vi "DrawRectangle.vi"() -> ()   [LabVIEW 2020]
panel:
  in  "path to BMP file":path
  out "2D Picture":picture
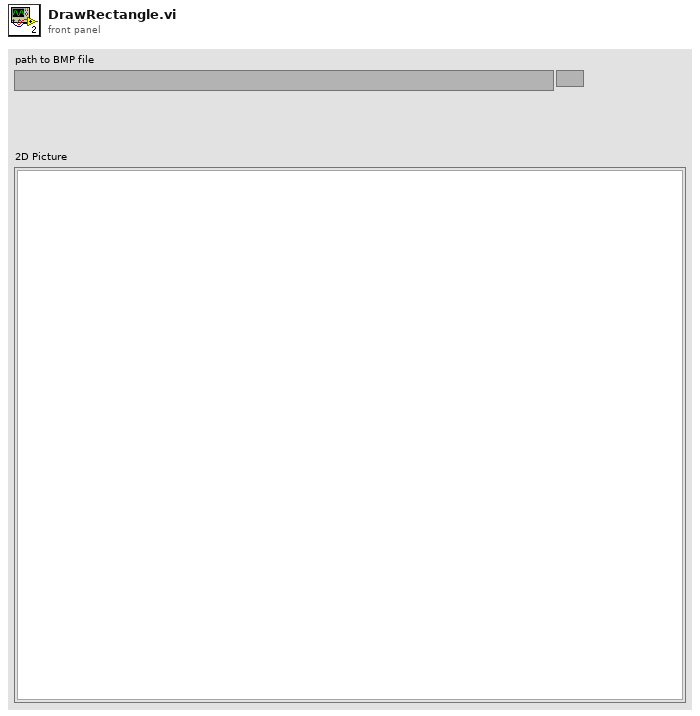
[diagram p1: front panel]
types:
  T1 = typedef "imagedata.ctl" = cluster{"image type":i32, "image depth":i32, "image":u8[], "mask":u8[], "colors":u32[], "Rectangle":cluster{"left":i16, "top":i16, "right":i16, "bottom":i16}}
  T2 = cluster{"Width":i16, "Style":enum32{"Solid", "Dash", "Dot", "DashDot", "DashDotDot"}}
  T3 = cluster{"left":i16, "top":i16, "right":i16, "bottom":i16}
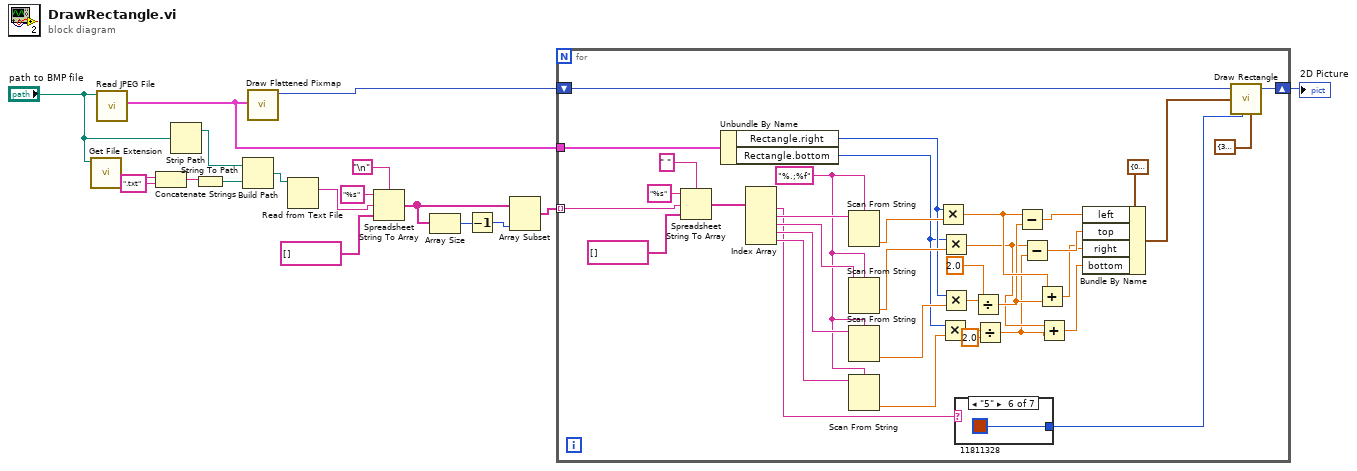
[diagram p0: block diagram]
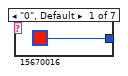
[diagram p2: hidden frame]
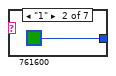
[diagram p3: hidden frame]
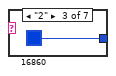
[diagram p4: hidden frame]
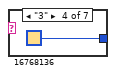
[diagram p5: hidden frame]
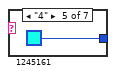
[diagram p6: hidden frame]
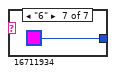
[diagram p7: hidden frame]
diagram:
  n1 = call <vilib>:"Get File Extension.vi"("file"="path to BMP file") -> ("filename without extension"=w18:string)  [unwired: 6 in, 4 out]
  n2 = call <vilib>:"Read JPEG File.vi"("path to JPEG file"="path to BMP file") -> ("image data"=w9:T1)  [unwired: 8 in, 2 out]
  n3 = Concatenate Strings(w18, ".txt" ("string")) -> (w16:string)
  n4 = Strip Path(path="path to BMP file") -> (stripped path=w13:path)  [unwired: 1 out]
  n5 = String To Path(string=w16) -> (path=w15:path)
  n6 = Build Path(base path=w13, name or relative path=w15) -> (appended path=w12:path)
  n7 = call <vilib>:"Draw Flattened Pixmap.vi"("image data"=w9) -> ("new picture"=w10:picture)  [unwired: 8 in]
  n8 = Read from Text File(file (use dialog)=w12) -> (text=w6:string)  [unwired: 3 in, 3 out]
  n9 = Spreadsheet String To Array(delimiter (Tab)="\n", format string="%s", spreadsheet string=w6, array type (2D Dbl)=string[] []) -> (array=w3:string[])
  n10 = Array Size(array=w3) -> (size(s)=w2:i32)
  n11 = Decrement(x=w2) -> (x-1=w1:i32)
  n12 = Array Subset(array=w3, length=w1) -> (w4:string[])  [unwired: 1 in]
  n13 = for {
    tunnel: w9 -> [w34]
    shift-right: [w39] -> w11
    shift-left: w10 -> [w35]
    tunnel: w4 -> [w20] mode=indexing
    w46 = "%.;%f" ("format string")
    n14 = Spreadsheet String To Array(delimiter (Tab)=" ", format string="%s", spreadsheet string=w20, array type (2D Dbl)=string[] []) -> (array=w52:string[])
    n15 = Unbundle By Name(w34) -> ("Rectangle.right"=w41:i16, "Rectangle.bottom"=w40:i16)
    n16 = Index Array(array=w52) -> (element #1=w19:string, element #2=w50:string, element #3=w47:string, element #4=w48:string, element #5=w49:string)  [unwired: 5 in]
    n17 = Scan From String(format string=w46, input string=w50) -> (output 1=w43:dbl)  [unwired: 3 in, 3 out]
    n18 = Scan From String(format string=w46, input string=w47) -> (output 1=w42:dbl)  [unwired: 3 in, 3 out]
    n19 = Scan From String(format string=w46, input string=w48) -> (output 1=w44:dbl)  [unwired: 3 in, 3 out]
    n20 = Scan From String(format string=w46, input string=w49) -> (output 1=w45:dbl)  [unwired: 3 in, 3 out]
    n21 = Multiply(x=w41, y=w43) -> (x*y=w27:dbl)
    n22 = Multiply(x=w40, y=w45) -> (x*y=w32:dbl)
    n23 = Multiply(x=w40, y=w42) -> (x*y=w24:dbl)
    n24 = Multiply(x=w41, y=w44) -> (x*y=w33:dbl)
    n25 = case shown="\"5\"" w19 {
      tunnel: [u32 15670016 ("color(black)") u32 761600 ("color(black)") u32 16860 ("color(black)") u32 16768136 ("color(black)") u32 1245161 ("color(black)") u32 11811328 ("color(black)") u32 16711934 ("color(black)")] -> w21
      frame "0", Default {
      }
      frame "1" {
      }
      frame "2" {
      }
      frame "3" {
      }
      frame "4" {
      }
      frame "5" {
      }
      frame "6" {
      }
    }
    n26 = Divide(x=w33, y=2.0) -> (x/y=w26:dbl)
    n27 = Divide(x=w32, y=2.0) -> (x/y=w23:dbl)
    n28 = Subtract(x=w27, y=w26) -> (x-y=w29:dbl)
    n29 = Subtract(x=w24, y=w23) -> (x-y=w28:dbl)
    n30 = Add(x=w27, y=w26) -> (x+y=w25:dbl)
    n31 = Add(x=w24, y=w23) -> (x+y=w22:dbl)
    n32 = Bundle By Name(cluster=T3 {"left"=0, "top"=0, "right"=0, "bottom"=0} ("rect"), "left"=w29, "top"=w28, "right"=w25, "bottom"=w22) -> (w37:T3)
    n33 = call <vilib>:"Draw Rectangle.vi"("picture"=w35, "rect"=w37, "color(black)"=w21, "pen"=T2 {"Width"=3, "Style"=enum."Solid"}) -> ("new picture"=w39:picture)  [unwired: 5 in]
  }
  "2D Picture" <- w11
